vi "getSelf.vi"() -> (0 "TestCase.lvclass":refnum<class "TestCase.lvclass">)   [LabVIEW 2019, in "TestCase.lvclass"]
uses:
  TestCase.lvclass
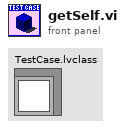
[diagram p1: front panel]
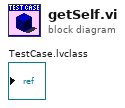
[diagram p0: block diagram]
diagram:
